vi "BulkRename.vi"() -> ()   [LabVIEW 2022 SP3]
uses:
  <vilib>/regexp/Match Regular Expression.xnode
panel:
  out "Progress":u8(slide) scale=0.0..100.0
  in  "Rename":bool
  out "Example New Name":string
  in  "Match Replacement":string
  in  "regular expression":string
  out "after match":string
  out "whole match":string
  out "before match":string
  out "Files":string[](array[string])
  in  "Cancel":bool
  in  "Path":path
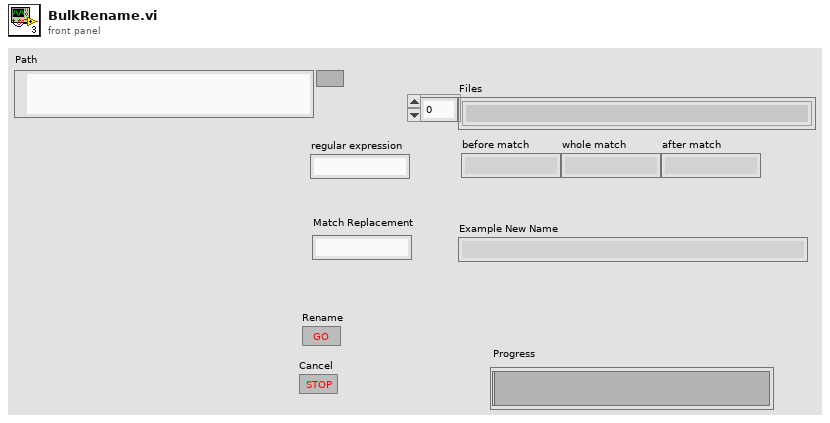
[diagram p1: front panel]
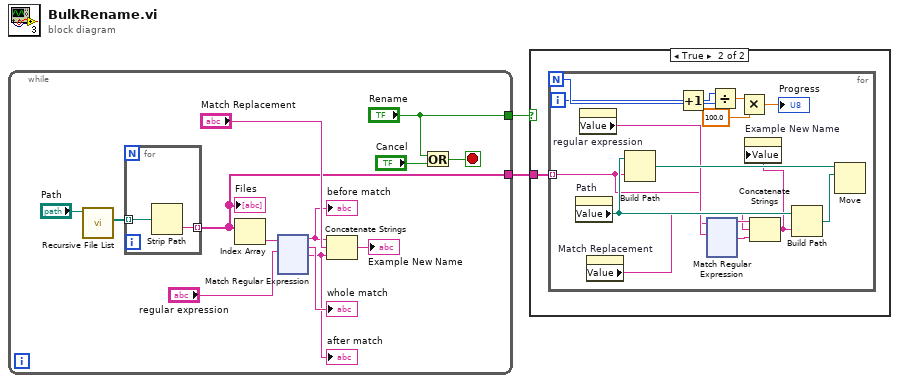
[diagram p0: block diagram]
diagram:
  n1 = while {
    tunnel: ["Rename"] -> w2
    tunnel: [w3] -> w1
    stop <- w5 stop-if-true
    n2 = call <vilib>:"Recursive File List.vi"("Folder Path"="Path") -> ("All Files in Dir"=w13:path[])  [unwired: 6 in, 4 out]
    n3 = for {
      tunnel: w13 -> [w134] mode=indexing
      tunnel: [w133] -> w3 mode=indexing
      n4 = Strip Path(path=w134) -> (name=w133:string)  [unwired: 1 out]
    }
    "Files" <- w3
    n5 = Index Array(array=w3) -> (element=w12:string)  [unwired: 1 in]
    n6 = xnode "Match Regular Expression"("input string"=w12, "regular expression"="regular expression") -> ("before match"=w8:string, "whole match"=→"whole match":string, "after match"=w7:string)  [unwired: 4 in, 2 out]
    "before match" <- w8
    "after match" <- w7
    n7 = Concatenate Strings(w8, "Match Replacement", w7) -> (→"Example New Name":string)
    n8 = Or(x="Rename", y="Cancel") -> (x .or. y?=w5:bool)
  }
  n9 = case shown="True" w2 {
    tunnel: w1 -> [_ w135]
    frame False {
    }
    frame True {
      n10 = for {
        N -> [w142]
        tunnel: w135 -> [w143] mode=indexing
        i -> [w141]
        n11 = property on="Path" class="Path"() -> ("Value"=w149:path)  [unwired: 2 in, 2 out]
        n12 = property on="regular expression" class="Str"() -> ("Value"=w144:string)  [unwired: 2 in, 2 out]
        n13 = property on="Match Replacement" class="Str"() -> ("Value"=w145:string)  [unwired: 2 in, 2 out]
        n14 = Build Path(base path=w149, name or relative path=w143) -> (appended path=w150:path)
        n15 = Increment(x=w141) -> (x+1=w140:i32)
        n16 = xnode "Match Regular Expression"("input string"=w143, "regular expression"=w144) -> ("before match"=w147:string, "after match"=w146:string)  [unwired: 4 in, 3 out]
        n17 = Divide(x=w140, y=w142) -> (x/y=w139:dbl)
        n18 = Multiply(x=w139, y=100.0) -> (x*y=→"Progress":dbl)
        n19 = Concatenate Strings(w147, w145, w146) -> (w136:string)
        n20 = property on="Example New Name" class="Str"("Value"=w136) -> ()  [unwired: 2 in, 2 out]
        n21 = Build Path(base path=w149, name or relative path=w136) -> (appended path=w148:path)
        n22 = Move(source path=w150, 10:w148) -> ()  [unwired: 3 in, 3 out]
      }
    }
  }
